vi "FlatToRichni_measurementlink_pinmap_v1_QueryResourceAccessInformationResponse_GroupMappingsEntry.vi"(5 "OutputClusterType":T1, 11 "InputCluster":T3) -> (3 "OutputCluster":T1)   [LabVIEW 2020, in "MeasurementLink Pin Map Client.lvlib"]
uses:
  MeasurementLink Pin Map Client.lvlib
  ni_measurementlink_pinmap_v1_QueryResourceAccessInformationResponse_GroupMappingsEntry_Flat.ctl
  ni_measurementlink_pinmap_v1_ResolvedPinsOrRelays_Flat.ctl
  ni_measurementlink_pinmap_v1_QueryResourceAccessInformationResponse_GroupMappingsEntry.ctl
  ni_measurementlink_pinmap_v1_ResolvedPinsOrRelays.ctl
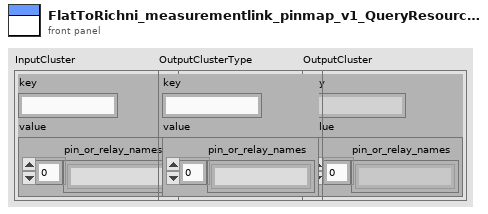
[diagram p1: front panel]
types:
  T1 = typedef "MeasurementLink Pin Map Client.lvlib/ni_measurementlink_pinmap_v1_QueryResourceAccessInformationResponse_GroupMappingsEntry.ctl" = cluster{"key":string, "value":T2}
  T2 = typedef "MeasurementLink Pin Map Client.lvlib/ni_measurementlink_pinmap_v1_ResolvedPinsOrRelays.ctl" = cluster{"pin_or_relay_names":string[]}
  T3 = typedef "MeasurementLink Pin Map Client.lvlib/ni_measurementlink_pinmap_v1_QueryResourceAccessInformationResponse_GroupMappingsEntry_Flat.ctl" = cluster{"key":string, "value":T4}
  T4 = typedef "MeasurementLink Pin Map Client.lvlib/ni_measurementlink_pinmap_v1_ResolvedPinsOrRelays_Flat.ctl" = cluster{"pin_or_relay_names":string[]}
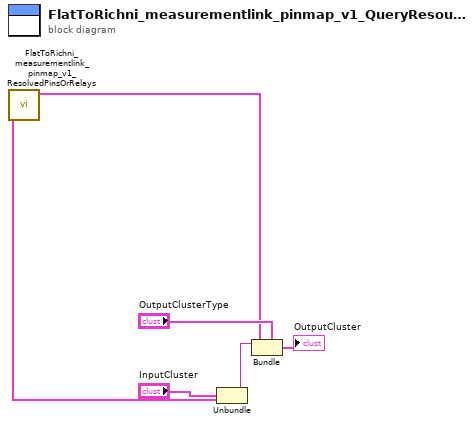
[diagram p0: block diagram]
diagram:
  n1 = Unbundle "Unbundle"("InputCluster") -> ("key"=w3:string, "value"=w2:T4)
  n2 = call "FlatToRichni_measurementlink_pinmap_v1_ResolvedPinsOrRelays.vi"("InputCluster"=w2) -> ("OutputCluster"=w1:T2)  [unwired: 10 in]
  n3 = Bundle "Bundle"(cluster="OutputClusterType", "key"=w3, "value"=w1) -> (→"OutputCluster":T1)
